vi "HopstitalFGV.vi"(7 "?":T1, 8 "error in (no error)":errorcluster, 9 "Room":i32, 10 "Flag In":bool[](array[boolean])) -> (0 "error out":errorcluster, 2 "Flag Out":bool[](array[boolean]))   [LabVIEW 2015]
uses:
  ActionEnum.ctl
  temp Room.ctl
  StateCluster.ctl
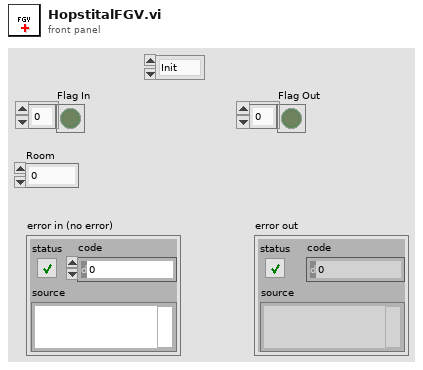
[diagram p1: front panel]
types:
  T1 = typedef "ActionEnum.ctl" = enum16{"Init", "Read", "Write"}
  T2 = typedef "StateCluster.ctl" = cluster{"Array":T3[]}
  T3 = typedef "temp Room.ctl" = cluster{"Flag":bool[]}
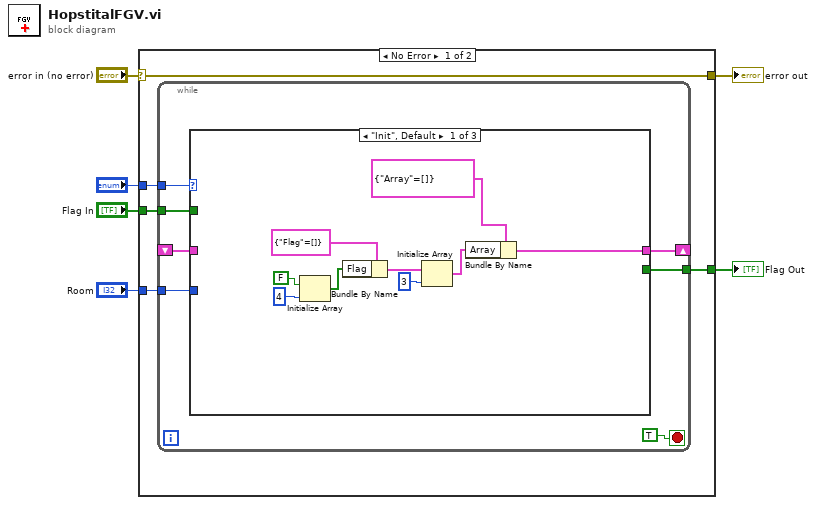
[diagram p0: block diagram]
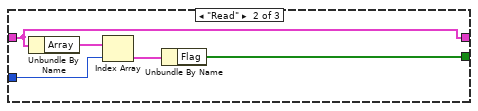
[diagram p2: hidden frame]
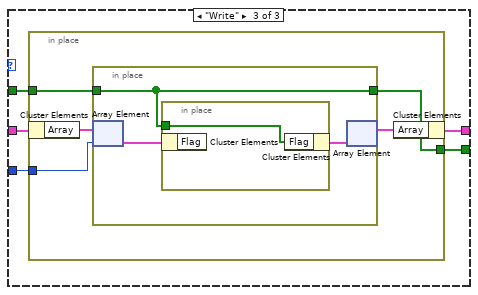
[diagram p3: hidden frame]
diagram:
  n1 = case shown="No Error" "error in (no error)" {
    selector: "error in (no error)" -> [w7 w47]
    tunnel: "?" -> [w11 _]
    tunnel: "Room" -> [w10 _]
    tunnel: [w9 _] -> w4
    tunnel: "Flag In" -> [w8 _]
    tunnel: [w7 w47] -> w1
    frame No Error {
      n2 = while {
        shift-right: [w16] -> _
        shift-left: _ -> [w15]
        tunnel: w11 -> [w17]
        tunnel: w10 -> [w14]
        tunnel: [w13] -> w9
        tunnel: w8 -> [w12]
        stop <- TRUE ("stop") stop-if-true
        n3 = case shown="\"Init\", Default" w17 {
          tunnel: [w26 w32 w36] -> w16
          tunnel: w15 -> [_ w32 w37]
          tunnel: w14 -> [_ w30 w34]
          tunnel: [_ w28 w33] -> w13
          tunnel: w12 -> [_ _ w35]
          frame "Init", Default {
            n4 = Initialize Array(FALSE ("element"), 4 ("dimension size")) -> (w24:bool[])
            n5 = Bundle By Name(cluster=T3 {"Flag"=[]} ("Room"), "Flag"=w24) -> (w21:T3)
            n6 = Initialize Array(w21, 3 ("dimension size")) -> (w20:T3[])
            n7 = Bundle By Name(cluster=T2 {"Array"=[]}, "Array"=w20) -> (w26:T2)
          }
          frame "Read" {
            n8 = Unbundle By Name(w32) -> ("Array"=w31:T3[])
            n9 = Index Array(array=w31, index=w30) -> (element=w29:T3)
            n10 = Unbundle By Name(w29) -> ("Flag"=w28:bool[])
          }
          frame "Write" {
            n11 = in-place {
              in-place-border: w35 -> [w42]
              in-place-border: w34 -> [w40]
              in-place-border: [w38] -> w33
              n12 = in-place-cluster #1(w37) -> ("Array"=w41:T3[])
              n13 = in-place {
                in-place-border: w42 -> [w43]
                in-place-border: [w43] -> w38
                n14 = in-place-array #2(w41, w40) -> (w45:T3)
                n15 = in-place {
                  in-place-border: w43 -> [w46]
                  n16 = in-place-cluster #3(w45) -> ()  [unwired: 1 out]
                  n17 = in-place-cluster #3("Flag"=w46) -> (w44:T3)
                }
                n18 = in-place-array #2(w44) -> (w39:T3[])  [unwired: 1 out]
              }
              n19 = in-place-cluster #1("Array"=w39) -> (w36:T2)
            }
          }
        }
      }
    }
    frame Error {
    }
  }
  "Flag Out" <- w4
  "error out" <- w1
